vi "Write Energy.vi"(8 "error in (no error)":errorcluster, 10 "Energy":i16=100, 11 "Nigel Tamagotchi in":refnum<class "Tamagotchi Basic Actor.lvclass">) -> (0 "error out":errorcluster, 3 "Nigel Tamagotchi out":refnum<class "Tamagotchi Basic Actor.lvclass">)   [LabVIEW 2026, in "Tamagotchi Basic Actor.lvclass"]
uses:
  Tamagotchi Basic Actor.lvclass
  Tamagotchi Basic Actor.lvclass/Tamagotchi Basic Actor.ctl
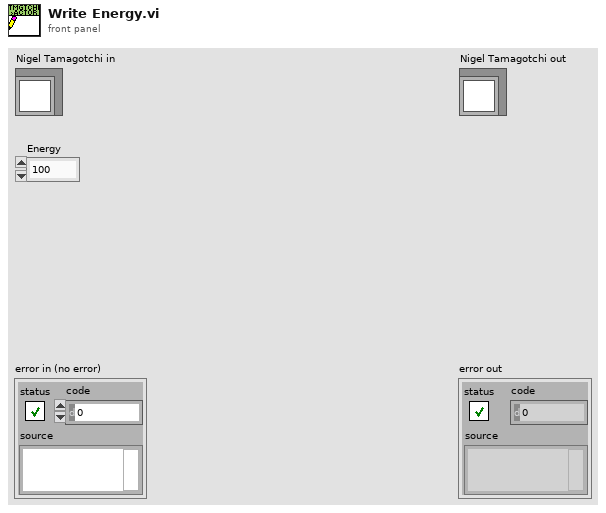
[diagram p1: front panel]
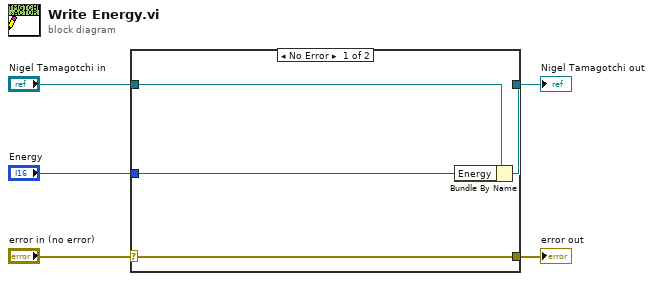
[diagram p0: block diagram]
diagram:
  n1 = case shown="No Error" "error in (no error)" {
    selector: "error in (no error)" -> [w9 w10]
    tunnel: [w9 w10] -> w4
    tunnel: [w7 w11] -> w2
    tunnel: "Nigel Tamagotchi in" -> [w8 w11]
    tunnel: "Energy" -> [w6 _]
    frame No Error {
      n2 = Bundle By Name(cluster=w8, "Energy"=w6) -> (w7:refnum<class "Tamagotchi Basic Actor.lvclass">)
    }
    frame Error {
    }
  }
  "error out" <- w4
  "Nigel Tamagotchi out" <- w2
